vi "frequencySweepAndReadSubVI.vi"(0 "file (use dialog)":path, 4 "Set Initial Frequency":string, 5 "Set GPIB":refnum<visa-resource-name>, 6 "Set Final Frequency":string, 8 "Set Increment":string, 10 "Time Delay (sec)":u32, 11 "error in (no error) 3":errorcluster) -> (1 "VX":string, 2 "VY":string, 3 "VR":string, 12 "Phase":string, 15 "Frequency":string)   [LabVIEW 2012]
uses:
  Global 1.vi
panel:
  out "concatenated string 2":string
  out "concatenated string":string
  out "error out 3":errorcluster
  out "error out":errorcluster
  in  "error in (no error) 2":errorcluster
  out "Increment":i32
  out "Final Frequency":i32
  out "Initial Frequency":i32
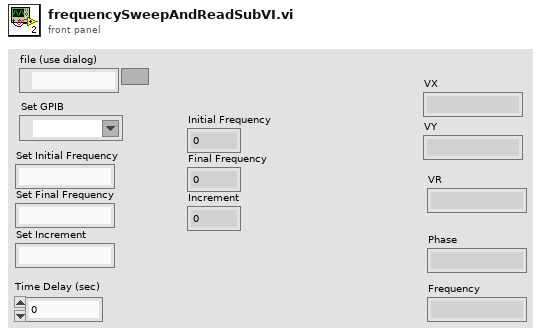
[diagram p1: front panel]
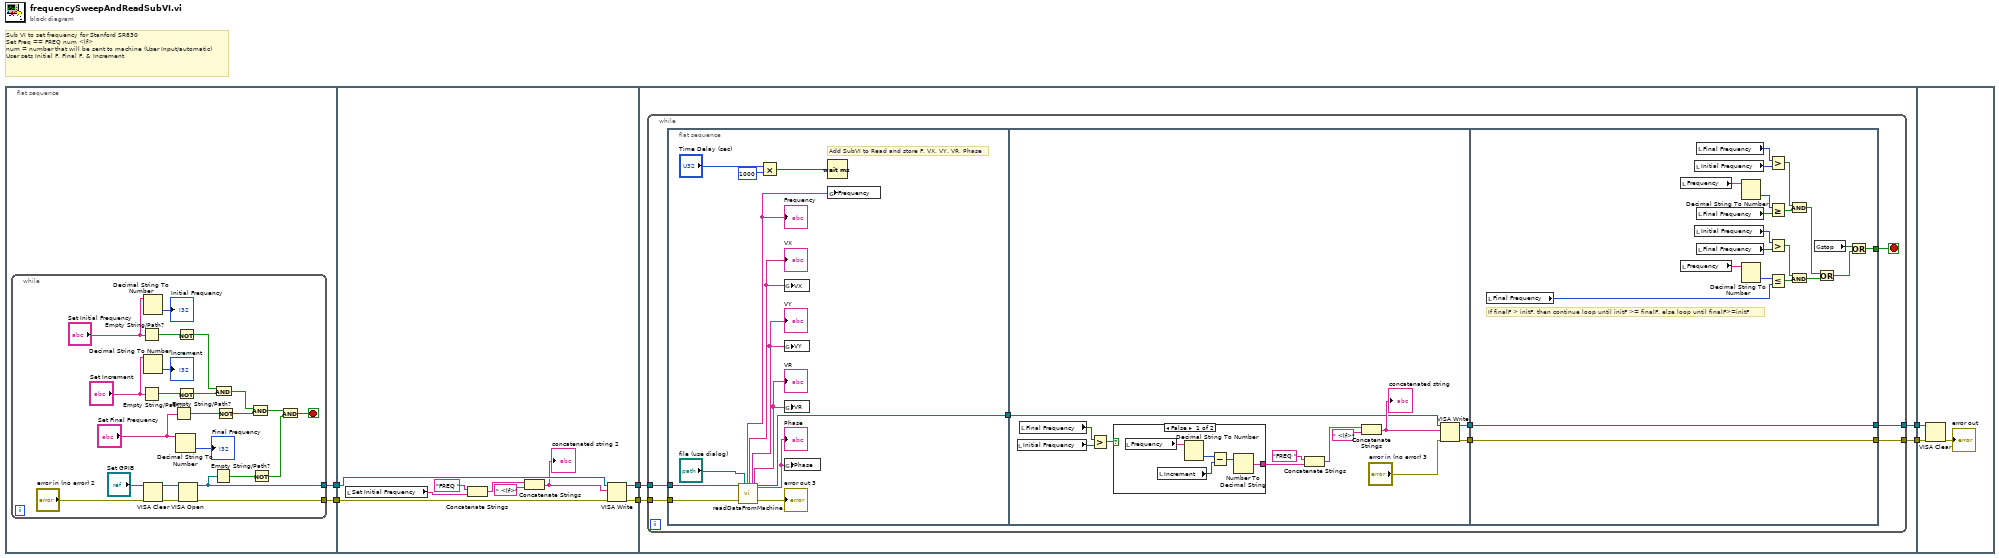
[diagram p0: block diagram]
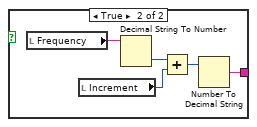
[diagram p2: hidden frame]
diagram:
  # "Sub VI to set frequency for Stanford SR830\nSet Freq == FREQ num <lf>\nnum = number that will be sent to machine (User Input/automatic)\nUser sets Initial F, Final F, & Increment"
  n1 = flat-sequence {
    tunnel: [w8] -> w6
    tunnel: [w7] -> w5
    tunnel: w6 -> [w40]
    tunnel: w5 -> [w39]
    tunnel: [w33] -> w4
    tunnel: [w32] -> w3
    tunnel: w4 -> [w44]
    tunnel: w3 -> [w43]
    tunnel: [w42] -> w2
    tunnel: [w41] -> w1
    tunnel: w2 -> [w110]
    tunnel: w1 -> [w111]
    frame #0 {
      n2 = while {
        tunnel: [w17] -> w8
        tunnel: [w18] -> w7
        stop <- w13 stop-if-true
        n3 = Empty String/Path?(string/path="Set Initial Frequency") -> (empty?=w27:bool)
        n4 = Empty String/Path?(string/path="Set Increment") -> (empty?=w24:bool)
        n5 = Decimal String To Number(string="Set Initial Frequency") -> (number=→"Initial Frequency":i32)  [unwired: 2 in, 1 out]
        n6 = Decimal String To Number(string="Set Increment") -> (number=→"Increment":i32)  [unwired: 2 in, 1 out]
        n7 = VISA Clear(VISA resource name="Set GPIB", error in (no error)="error in (no error) 2") -> (VISA resource name out=w9:refnum<visa-resource-name>, error out=w11:errorcluster)
        n8 = Empty String/Path?(string/path="Set Final Frequency") -> (empty?=w21:bool)
        n9 = Decimal String To Number(string="Set Final Frequency") -> (number=→"Final Frequency":i32)  [unwired: 2 in, 1 out]
        n10 = Not(x=w27) -> (.not. x?=w26:bool)
        n11 = Not(x=w24) -> (.not. x?=w23:bool)
        n12 = VISA Open(error in (no error)=w11, VISA resource name=w9) -> (VISA resource name=w17:refnum<visa-resource-name>, error out=w18:errorcluster)  [unwired: 3 in]
        n13 = Empty String/Path?(string/path=w17) -> (empty?=w16:bool)
        n14 = And(x=w26, y=w23) -> (x .and. y?=w19:bool)
        n15 = Not(x=w21) -> (.not. x?=w20:bool)
        n16 = And(x=w19, y=w20) -> (x .and. y?=w15:bool)
        n17 = Not(x=w16) -> (.not. x?=w14:bool)
        n18 = And(x=w15, y=w14) -> (x .and. y?=w13:bool)
      }
    }
    frame #1 {
      n19 = local read "Set Initial Frequency"() -> (w37:string)
      n20 = Concatenate Strings("FREQ " ("string"), w37) -> (w36:string)
      n21 = Concatenate Strings(w36, " <lf>" ("string")) -> (w34:string)
      "concatenated string 2" <- w34
      n22 = VISA Write(VISA resource name=w40, write buffer=w34, error in (no error)=w39) -> (VISA resource name out=w32:refnum<visa-resource-name>, error out=w33:errorcluster)  [unwired: 1 out]
    }
    frame #2 {
      n23 = while {
        tunnel: w44 -> [w52]
        tunnel: w43 -> [w51]
        tunnel: [w50] -> w42
        tunnel: [w48] -> w41
        stop <- w45 stop-if-true
        n24 = flat-sequence {
          tunnel: w52 -> [w61]
          tunnel: w51 -> [w62]
          tunnel: [w59] -> w46
          tunnel: [w73] -> w49
          tunnel: [w72] -> w47
          tunnel: w46 -> [w66]
          tunnel: [w88] -> w45
          tunnel: [w92] -> w50
          tunnel: w49 -> [w92]
          tunnel: [w91] -> w48
          tunnel: w47 -> [w91]
          frame #0 {
            # "Add SubVI to Read and store F, VX, VY, VR, Phase"
            n25 = call "readDataFromMachine.vi"("VISA resource name"=w62, "error in (no error)"=w61, "file (use dialog)"="file (use dialog)") -> ("Frequency"=w54:string, "VX"=w56:string, "VY"=w57:string, "VR"=w55:string, "VISA resource name out"=w59:refnum<visa-resource-name>, "Phase"=w53:string, "error out"=→"error out 3":errorcluster)  [unwired: 17 in, 1 out]
            "VX" <- w56
            "VY" <- w57
            "VR" <- w55
            "Frequency" <- w54
            "Phase" <- w53
            n26 = Multiply(x="Time Delay (sec)", y=u32 1000) -> (x*y=w63:u32)
            n27 = global write "Global 1.vi" "VX"(w56) -> ()
            n28 = global write "Global 1.vi" "VY"(w57) -> ()
            n29 = global write "Global 1.vi" "VR"(w55) -> ()
            n30 = global write "Global 1.vi" "Phase"(w53) -> ()
            n31 = Wait (ms)(milliseconds to wait=w63) -> ()  [unwired: 1 out]
            n32 = global write "Global 1.vi" "Frequency"(w54) -> ()
          }
          frame #1 {
            n33 = local read "Initial Frequency"() -> (w69:i32)
            n34 = local read "Final Frequency"() -> (w70:i32)
            n35 = Greater?(x=w70, y=w69) -> (0:w68:bool)
            n36 = case shown="False" w68 {
              tunnel: [w78 w83] -> w71
              frame False {
                n37 = local read "Frequency"() -> (w82:string)
                n38 = local read "Increment"() -> (w80:i32)
                n39 = Decimal String To Number(string=w82) -> (number=w81:i32)  [unwired: 2 in, 1 out]
                n40 = Subtract(x=w81, y=w80) -> (x-y=w79:i32)
                n41 = Number To Decimal String(number=w79) -> (decimal integer string=w78:string)  [unwired: 1 in]
              }
              frame True {
                n42 = local read "Frequency"() -> (w87:string)
                n43 = local read "Increment"() -> (w85:i32)
                n44 = Decimal String To Number(string=w87) -> (number=w86:i32)  [unwired: 2 in, 1 out]
                n45 = Add(x=w86, y=w85) -> (x+y=w84:i32)
                n46 = Number To Decimal String(number=w84) -> (decimal integer string=w83:string)  [unwired: 1 in]
              }
            }
            n47 = Concatenate Strings("FREQ " ("string"), w71) -> (w76:string)
            n48 = Concatenate Strings(w76, " <lf>" ("string")) -> (w74:string)
            "concatenated string" <- w74
            n49 = VISA Write(VISA resource name=w66, write buffer=w74, error in (no error)="error in (no error) 3") -> (VISA resource name out=w72:refnum<visa-resource-name>, error out=w73:errorcluster)  [unwired: 1 out]
          }
          frame #2 {
            # "If finalF > initF, then continue loop until initF >= finalF, else loop until finalF>=initF"
            n50 = local read "Final Frequency"() -> (w95:i32)
            n51 = local read "Frequency"() -> (w105:string)
            n52 = local read "Frequency"() -> (w97:string)
            n53 = local read "Initial Frequency"() -> (w107:i32)
            n54 = local read "Initial Frequency"() -> (w100:i32)
            n55 = local read "Final Frequency"() -> (w108:i32)
            n56 = local read "Final Frequency"() -> (w103:i32)
            n57 = local read "Final Frequency"() -> (w99:i32)
            n58 = Decimal String To Number(string=w105) -> (number=w104:i32)  [unwired: 2 in, 1 out]
            n59 = Decimal String To Number(string=w97) -> (number=w96:i32)  [unwired: 2 in, 1 out]
            n60 = Greater?(x=w108, y=w107) -> (0:w106:bool)
            n61 = Greater Or Equal?(x=w104, y=w103) -> (x >= y?=w102:bool)
            n62 = Greater?(x=w100, y=w99) -> (0:w98:bool)
            n63 = Less Or Equal?(x=w96, y=w95) -> (x <= y?=w94:bool)
            n64 = And(x=w106, y=w102) -> (x .and. y?=w101:bool)
            n65 = And(x=w98, y=w94) -> (x .and. y?=w93:bool)
            n66 = global read "Global 1.vi" "stop"() -> (w90:bool)
            n67 = Or(x=w101, y=w93) -> (x .or. y?=w89:bool)
            n68 = Or(x=w90, y=w89) -> (x .or. y?=w88:bool)
          }
        }
      }
    }
    frame #3 {
      n69 = VISA Clear(VISA resource name=w111, error in (no error)=w110) -> (error out=→"error out":errorcluster)  [unwired: 1 out]
    }
  }
